vi "UIRefs Desired Gas.vi"(8 "error in (no error)":errorcluster, 11 "FC2901 in":refnum<class "FC2901.lvclass">) -> (0 "error out":errorcluster, 3 "FC2901 out":refnum<class "FC2901.lvclass">)   [LabVIEW 2021, in "FC2901.lvclass"]
uses:
  FC2901.lvclass
  FC2901.lvclass/FC2901.ctl
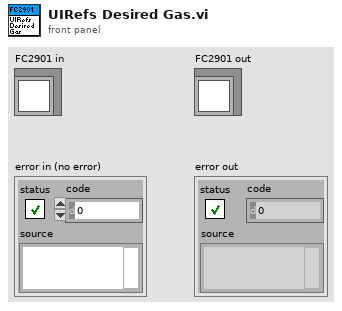
[diagram p1: front panel]
types:
  T1 = typedef "C100L.lvclass/GCF Data.ctl" = map{string, dbl}
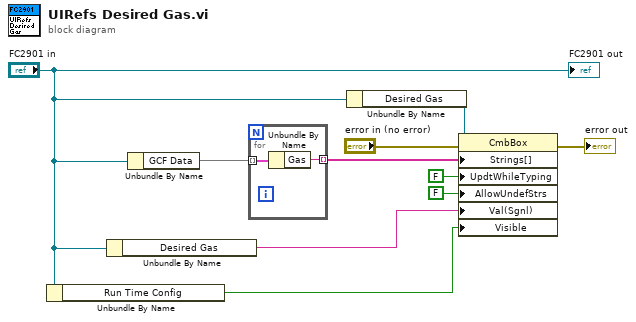
[diagram p0: block diagram]
diagram:
  n1 = Unbundle By Name("FC2901 in") -> ("Run Time Config"=w1:bool)
  n2 = Unbundle By Name("FC2901 in") -> ("Desired Gas"=w3:string)
  n3 = Unbundle By Name("FC2901 in") -> ("GCF Data"=w9:T1)
  n4 = for {
    tunnel: [w11] -> w6 mode=indexing
    tunnel: w9 -> [w12] mode=indexing
    n5 = Unbundle By Name(w12) -> ("Gas"=w11:string)
  }
  n6 = Unbundle By Name("FC2901 in") -> ("Desired Gas"=w10:refnum<vi>)
  n7 = property class="CmbBox"(reference=w10, error in="error in (no error)", "Strings[]"=w6, "UpdtWhileTyping"=FALSE ("Update While Typing?"), "AllowUndefStrs"=FALSE ("Allow Undefined Strings"), "Val(Sgnl)"=w3, "Visible"=w1) -> (error out=→"error out":errorcluster)  [unwired: 1 out]
  "FC2901 out" <- "FC2901 in"
